vi "Send GMail.vi"(5 "Password":string="LNip9102qwer$", 7 "Username":string="henslewm", 8 "error in":errorcluster, 9 "Message":string, 10 "Subject":string, 11 "To:":string[](array[string])) -> (0 "error out":errorcluster)   [LabVIEW 2014]
doc: "Uses the SMTP Email Client to send an email to a standard or secure SMTP server."
uses:
  <vilib>/smtpClient/SmtpClientHandle.ctl
  <vilib>/smtpClient/Set Message Text.vi
  <vilib>/smtpClient/LabVIEWSMTPClient.lvlib
panel:
  out "E-mail Destinations":i32
  # "Compose Email"
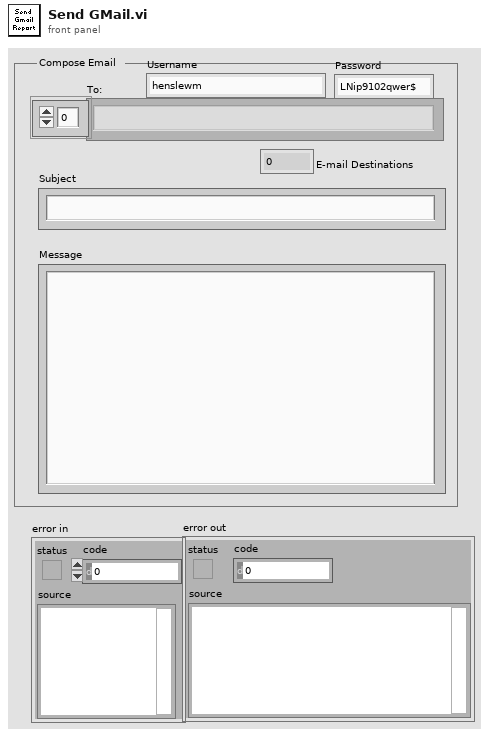
[diagram p1: front panel]
types:
  T1 = typedef "LabVIEWSMTPClient.lvlib/SmtpClientHandle.ctl" = refnum<k1>
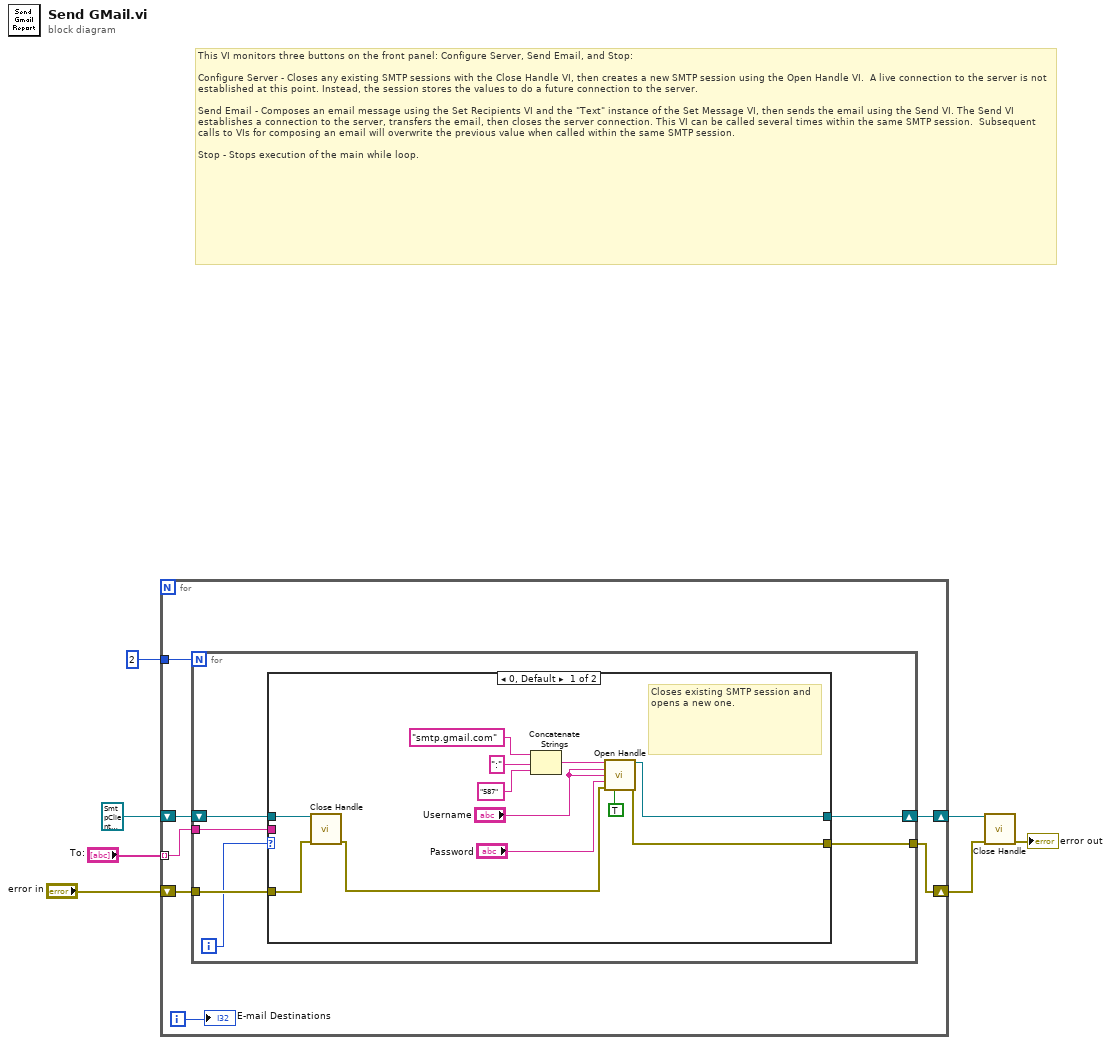
[diagram p0: block diagram]
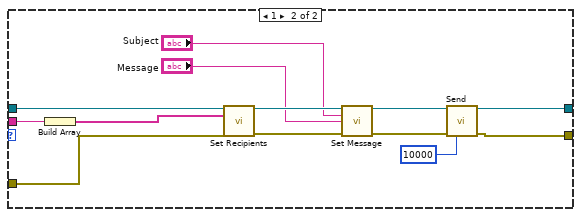
[diagram p2: hidden frame]
diagram:
  # "This VI monitors three buttons on the front panel: Configure Server, Send Email, and Stop:\n\nConfigure Server - Closes any existing SMTP sessions with the Close Handle VI, then creates a new SMTP session using the Open Handle VI.  A live connection to the server is not established at this point. Instead, the session stores the values to do a future connection to the server.\n\nSend Email - Composes an email message using the Set Recipients VI and the \"Text\" instance of the Set Message VI, then sends the email using the Send VI. The Send VI establishes a connection to the server, transfers the email, then closes the server connection. This VI can be called several times within the same SMTP session.  Subsequent calls to VIs for composing an email will overwrite the previous value when called within the same SMTP session.\n\nStop - Stops execution of the main while loop."
  n1 = for {
    tunnel: 2 -> [w10]
    shift-right: [w13] -> w5
    shift-left: T1 refnum ("handle out") -> [w14]
    shift-right: [w11] -> w3
    shift-left: "error in" -> [w12]
    tunnel: "To:" -> [w9] mode=indexing
    i -> [w8]
    n2 = for {
      N: w10 -> [_]
      shift-right: [w20] -> w13
      shift-left: w14 -> [w18]
      tunnel: w12 -> [w19]
      tunnel: [w17] -> w11
      tunnel: w9 -> [w15]
      i -> [w16]
      n3 = case shown="0, Default" w16 {
        tunnel: [w26 w35] -> w20
        tunnel: [w25 w36] -> w17
        tunnel: w19 -> [w23 w37]
        tunnel: w18 -> [w24 w38]
        tunnel: w15 -> [_ w34]
        frame 0, Default {
          # "Closes existing SMTP session and opens a new one."
          n4 = call <vilib>:"Close Handle.vi"("handle in"=w24, "error in (no error)"=w23) -> ("error out"=w22:errorcluster)  [unwired: 12 in, 1 out]
          n5 = Concatenate Strings("smtp.gmail.com" ("Outgoing Mail Server (SMTP)"), ":" ("string"), "587" ("Port")) -> (w29:string)
          n6 = call <vilib>:"Open Handle.vi"("server address"=w29, "from"="Username", "username"="Username", "password"="Password", "error in (no error)"=w22, "use TLS (false)"=TRUE ("Enable TLS")) -> ("handle out"=w26:T1, "error out"=w25:errorcluster)  [unwired: 8 in]
        }
        frame 1 {
          n7 = Build Array(w34) -> (w33:string[])
          n8 = call <vilib>:"Set Recipients.vi"("handle in"=w38, "to"=w33, "error in (no error)"=w37) -> ("handle out"=w42:T1, "error out"=w39:errorcluster)  [unwired: 11 in]
          n9 = call-poly <vilib>:"Set Message.vi"("handle in"=w42, "subject"="Subject", "plain text message"="Message", "error in (no error)"=w39) -> ("handle out"=w44:T1, "error out"=w43:errorcluster)  [unwired: 10 in]
          n10 = call <vilib>:"Send.vi"("handle in"=w44, "error in (no error)"=w43, "timeout in ms (10000)"=10000 ("timeout in ms")) -> ("handle out"=w35:T1, "error out"=w36:errorcluster)  [unwired: 10 in, 1 out]
        }
      }
    }
    "E-mail Destinations" <- w8
  }
  n11 = call <vilib>:"Close Handle.vi"("handle in"=w5, "error in (no error)"=w3) -> ("error out"=→"error out":errorcluster)  [unwired: 12 in, 1 out]
